vi "LWXPS_GetVarXSecondary.vi"(0 "XPS Reference IN":refnum<k24>, 5 "Name Parameter":string, 11 "LabVIEW error IN":errorcluster) -> (4 "XPS Reference OUT":refnum<k24>, 6 "Returned error code":i32, 8 "Value":dbl, 10 "XPS Error String":string, 15 "LabVIEW error OUT":errorcluster)   [LabVIEW 2014]
uses:
  D:/XPSQ8_LabView_Library/Development/Source/Dll/Newport.XPS.CommandInterface.dll
  Dll/Newport.XPS.CommandInterface.dll
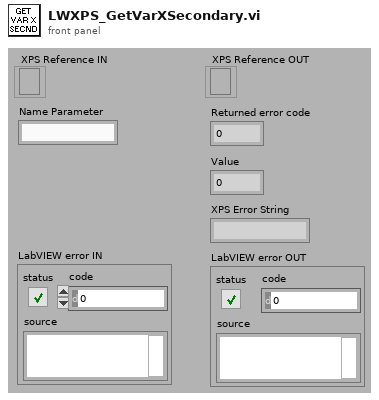
[diagram p1: front panel]
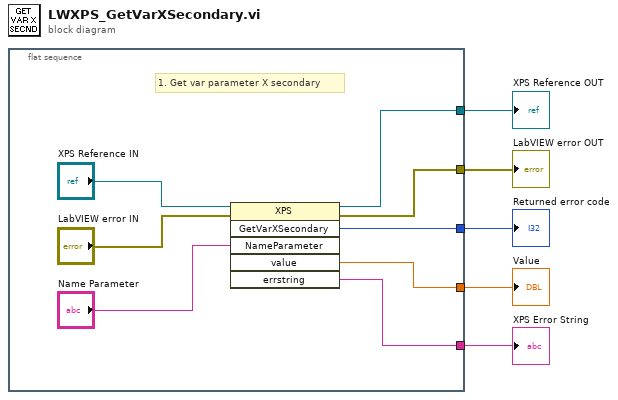
[diagram p0: block diagram]
diagram:
  n1 = flat-sequence {
    tunnel: [w6] -> w5
    tunnel: [w12] -> w4
    tunnel: [w10] -> w3
    tunnel: [w9] -> w2
    tunnel: [w8] -> w1
    frame #0 {
      # "1. Get var parameter X secondary"
      n2 = invoke class="XPS" method="GetVarXSecondary"(reference="XPS Reference IN", error in="LabVIEW error IN", "NameParameter"="Name Parameter") -> (reference out=w6:refnum<k24>, error out=w12:errorcluster, "GetVarXSecondary"=w10:i32, "value"=w9:dbl, "errstring"=w8:string)  [unwired: 3 in, 1 out]
    }
  }
  "XPS Reference OUT" <- w5
  "LabVIEW error OUT" <- w4
  "Returned error code" <- w3
  "Value" <- w2
  "XPS Error String" <- w1
